vi "Log Text.vi"(5 "csv/eco":bool, 7 "Log Array":string[](array[string]), 8 "error in (no error)":errorcluster caption="错误输入（无错误）", 9 "Hearder":string[](array[string]), 10 "log text":string, 11 "Path":path) -> (0 "error out":errorcluster caption="错误输出", 3 "standard output":string caption="标准输出")   [LabVIEW 2014]
uses:
  <vilib>/Utility/file.llb/Write Delimited Spreadsheet (string).vi
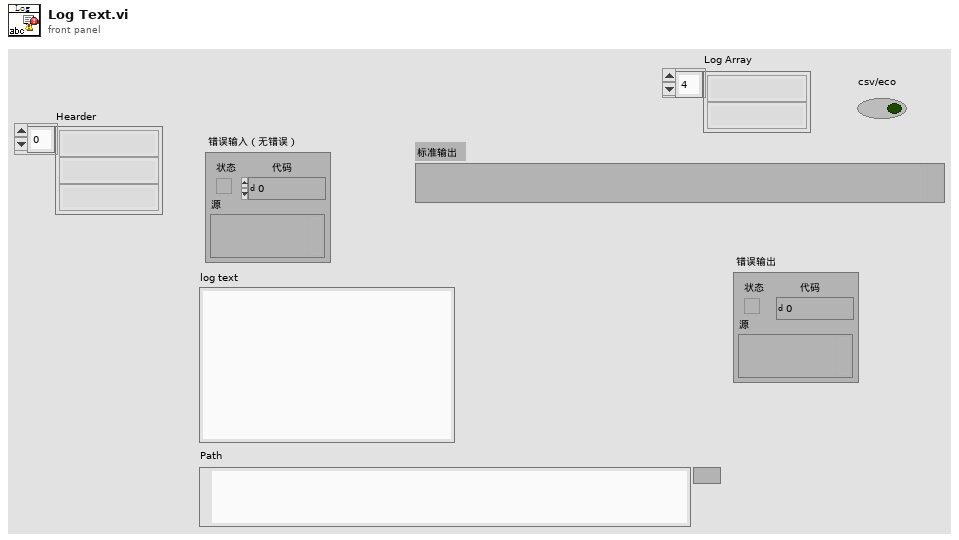
[diagram p1: front panel]
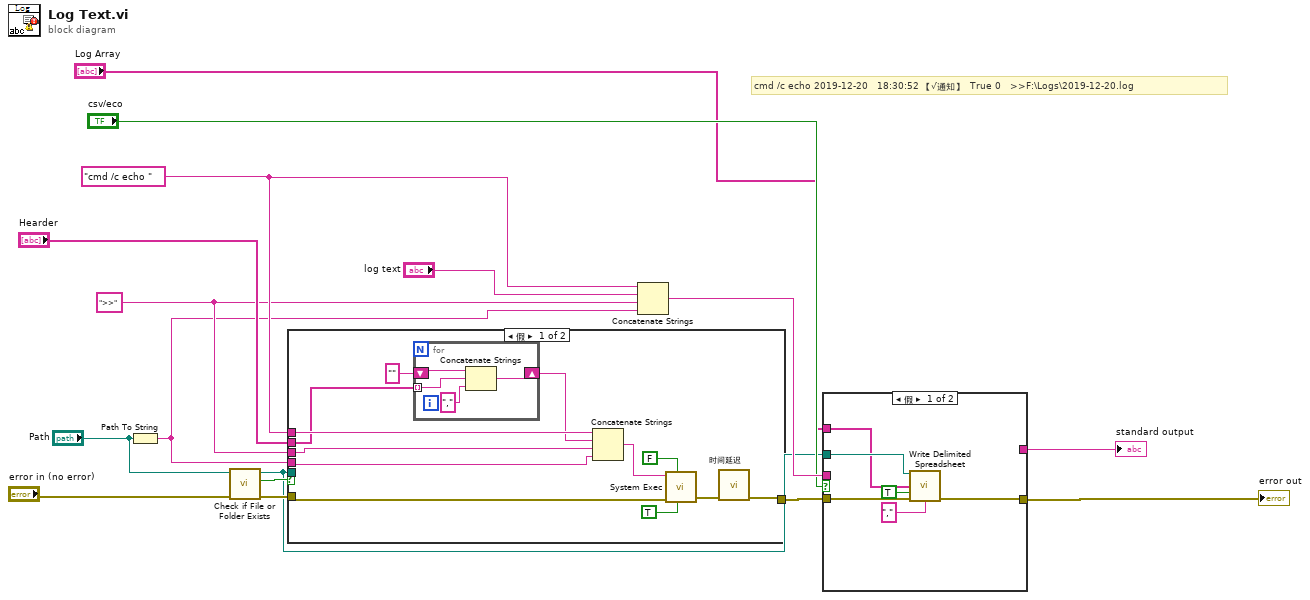
[diagram p0: block diagram]
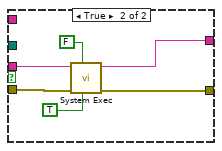
[diagram p2: hidden frame]
diagram:
  w7 = "cmd /c echo " ("command line")
  w5 = ">>"
  # "cmd /c echo 2019-12-20   18:30:52\t【√通知】\t\tTrue\t0\t\t >>F:\\Logs\\2019-12-20.log"
  n1 = Path To String(path="Path") -> (string=w4:string)
  n2 = call <vilib>:"Check if File or Folder Exists.vi"("error in (no error)"="error in (no error)", "path"="Path") -> ("error out"=w11:errorcluster, "file or folder exists?"=w10:bool, "dup path"=w2:path)  [unwired: 7 in]
  n3 = case shown="假" w10 {
    tunnel: w11 -> [w28 w33]
    tunnel: w2 -> [_ _]
    tunnel: [w22 w33] -> w8
    tunnel: w7 -> [w25 _]
    tunnel: "Hearder" -> [w20 _]
    tunnel: w5 -> [w24 _]
    tunnel: w4 -> [w17 _]
    frame False {
      n4 = for {
        shift-right: [w31] -> w19
        shift-left: "" -> [w32]
        tunnel: w20 -> [w30] mode=indexing
        n5 = Concatenate Strings(w32, w30, ",") -> (w31:string)
      }
      n6 = Concatenate Strings(w25, w19, w24, w17) -> (w18:string)
      n7 = call <vilib>:"System Exec.vi"("run minimized? (F)"=TRUE, "wait until completion? (T)"=FALSE, "error in (no error)"=w28, "command line"=w18) -> ("error out"=w23:errorcluster)  [unwired: 4 in, 3 out]
      n8 = call "时间延迟"("error in (no error)"=w23) -> ("error out"=w22:errorcluster)  [unwired: 10 in]
    }
    frame True {
    }
  }
  n9 = Concatenate Strings(w7, "log text", w5, w4) -> (w9:string)
  n10 = case shown="假" "csv/eco" {
    tunnel: [w38 w43] -> w16
    tunnel: [_ w42] -> w14
    tunnel: w9 -> [_ w41]
    tunnel: w8 -> [w39 w40]
    tunnel: w2 -> [w37 _]
    tunnel: "Log Array" -> [w36 _]
    frame False {
      n11 = call-poly <vilib>:"Write Delimited Spreadsheet.vi"("file path (dialog if empty)"=w37, "1D data"=w36, "append to file? (new file:F)"=TRUE, "error in (no error)"=w39, "delimiter (\\t)"="," ("delimiter (\\t)")) -> ("error out"=w38:errorcluster)  [unwired: 9 in, 1 out]
    }
    frame True {
      n12 = call <vilib>:"System Exec.vi"("run minimized? (F)"=TRUE, "wait until completion? (T)"=FALSE, "error in (no error)"=w40, "command line"=w41) -> ("error out"=w43:errorcluster, "standard output"=w42:string)  [unwired: 4 in, 2 out]
    }
  }
  "error out" <- w16
  "standard output" <- w14
